vi "T2.vi"(8 "error in (no error)":errorcluster, 11 "VISA Refnum in":refnum<visa-resource-name>) -> (0 "error out":errorcluster, 2 "Numeric":dbl, 3 "VISA Refnum out":refnum<visa-resource-name>)   [LabVIEW 2020]
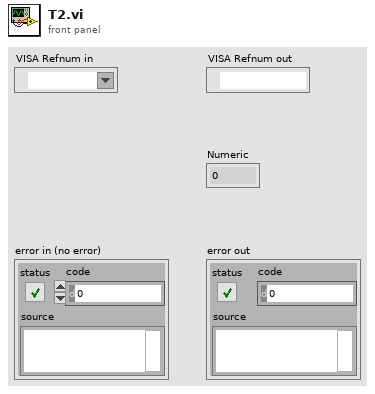
[diagram p1: front panel]
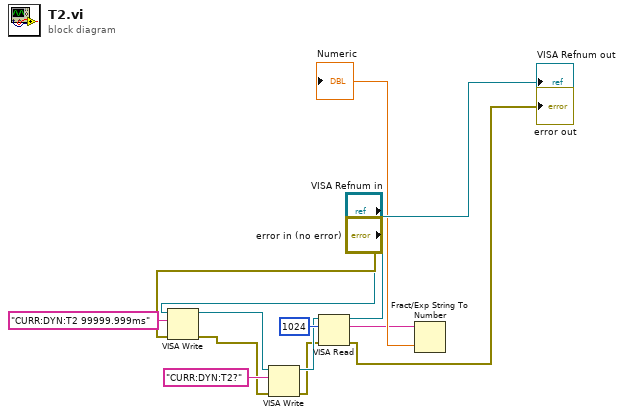
[diagram p0: block diagram]
diagram:
  n1 = VISA Write(VISA resource name="VISA Refnum in", write buffer="CURR:DYN:T2 99999.999ms", error in (no error)="error in (no error)") -> (VISA resource name out=w4:refnum<visa-resource-name>, error out=w2:errorcluster)  [unwired: 1 out]
  n2 = VISA Write(VISA resource name=w4, write buffer="CURR:DYN:T2?", error in (no error)=w2) -> (VISA resource name out=w3:refnum<visa-resource-name>, error out=w1:errorcluster)  [unwired: 1 out]
  n3 = VISA Read(VISA resource name=w3, byte count=u32 1024, error in (no error)=w1) -> (VISA resource name out=→"VISA Refnum out":refnum<visa-resource-name>, read buffer=w6:string, error out=→"error out":errorcluster)  [unwired: 1 out]
  n4 = Fract/Exp String To Number(string=w6) -> (number=→"Numeric":dbl)  [unwired: 3 in, 1 out]
